vi "divide matriz en submatrices.vi"(9 "Resolución":i32, 11 "Matriz compleja  A":T1) -> (0 "Número de elementos Vector C":i32, 1 "Vector C":cdb[][][][](array[numeric]) caption="Array", 2 "Vector B":cdb[][][](array[numeric]), 3 "Matriz compleja  A 2":T1)   [LabVIEW 2025]
uses:
  <vilib>/Analysis/Matrix/Datatypes/ComplexMatrix.ctl
  <vilib>/Analysis/Matrix/NI_Matrix.lvlib
panel:
  out "size(s)":i32[](array[numeric])
  out "number of rows":i32
  out "Número de matrices de cada elemento":i32
  out "No. filas":i32
  out "No. columnas":i32
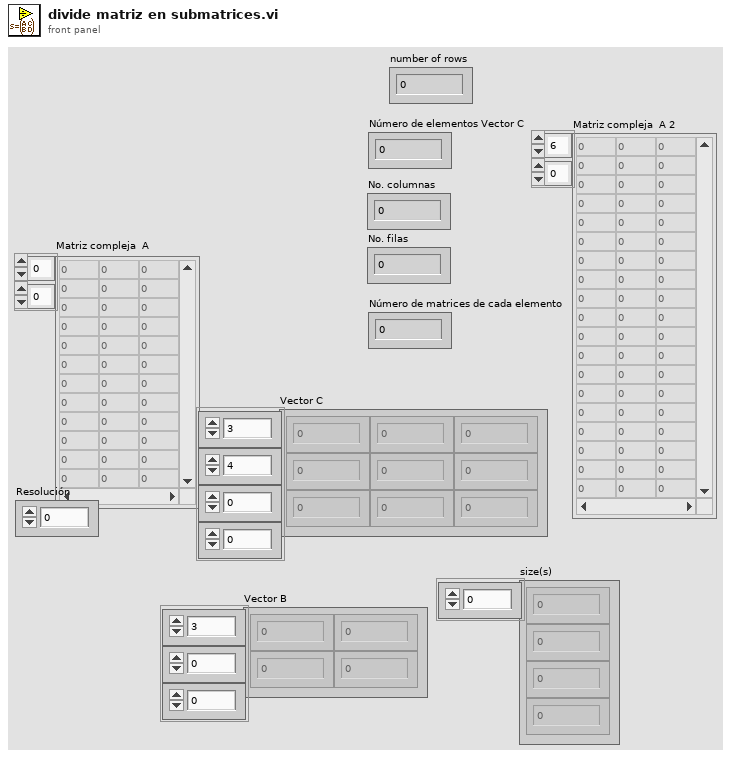
[diagram p1: front panel]
types:
  T1 = typedef "NI_Matrix.lvlib/ComplexMatrix.ctl" = cdb[][]
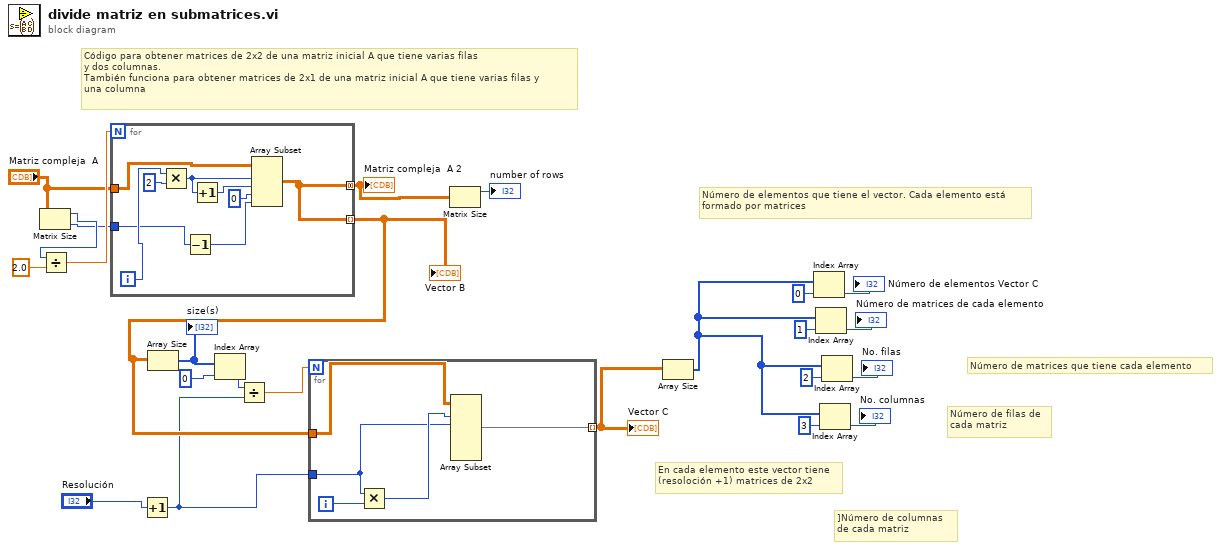
[diagram p0: block diagram]
diagram:
  # "]Número de columnas\nde cada matriz"
  # "Número de filas de\ncada matriz"
  # "Número de matrices que tiene cada elemento"
  # "Número de elementos que tiene el vector. Cada elemento está\nformado por matrices"
  # "En cada elemento este vector tiene\n(resoloción +1) matrices de 2x2"
  # "Código para obtener matrices de 2x2 de una matriz inicial A que tiene varias filas\ny dos columnas.\nTambién funciona para obtener matrices de 2x1 de una matriz inicial A que tiene varias filas y \nuna columna"
  n1 = Matrix Size(0:"Matriz compleja  A") -> (1:w23:i32, 2:w20:i32)
  n2 = Divide(x=w23, y=2.0) -> (x/y=w22:dbl)
  n3 = for {
    N: w22 -> [_]
    tunnel: "Matriz compleja  A" -> [w33]
    tunnel: w20 -> [w27]
    tunnel: [w25] -> w15 mode=indexing
    tunnel: [w25] -> w4 mode=concatenating
    i -> [w32]
    n4 = Multiply(x=w32, y=2) -> (x*y=w30:i32)
    n5 = Decrement(x=w27) -> (x-1=w26:i32)
    n6 = Increment(x=w30) -> (x+1=w29:i32)
    n7 = Array Subset(array=w33, index (row)=w30, length (row)=w29, index (col)=0 ("column 1"), length (col)=w26) -> (w25:T1)
  }
  "Vector B" <- w15
  "Matriz compleja  A 2" <- w4
  n8 = Increment(x="Resolución") -> (x+1=w1:i32)
  n9 = Array Size(array=w15) -> (size(s)=w19:i32[])
  "size(s)" <- w19
  n10 = Index Array(array=w19, index=0) -> (element=w17:i32)
  n11 = Divide(x=w17, y=w1) -> (x/y=w16:dbl)
  n12 = for {
    N: w16 -> [_]
    tunnel: w15 -> [w37]
    tunnel: [w35] -> w14 mode=indexing
    tunnel: w1 -> [w34]
    i -> [w38]
    n13 = Multiply(x=w34, y=w38) -> (x*y=w36:i32)
    n14 = Array Subset(array=w37, index (dim 0)=w36, length (dim 0)=w34) -> (w35:cdb[][][])  [unwired: 4 in]
  }
  "Vector C" <- w14
  n15 = Matrix Size(0:w4) -> (1:→"number of rows":i32)  [unwired: 1 out]
  n16 = Array Size(array=w14) -> (size(s)=w9:i32[])
  n17 = Index Array(array=w9, index=0) -> (element=→"Número de elementos Vector C":i32)
  n18 = Index Array(array=w9, index=1) -> (element=→"Número de matrices de cada elemento":i32)
  n19 = Index Array(array=w9, index=3) -> (element=→"No. columnas":i32)
  n20 = Index Array(array=w9, index=2) -> (element=→"No. filas":i32)
